vi "Send Trigger.vi"(8 "error in (no error)":errorcluster, 10 "Trigger Type (0: Bus)":u16(ring) items=["Bus", "Immediate"], 11 "VISA resource name":refnum<visa-resource-name>) -> (0 "error out":errorcluster, 3 "VISA resource name out":refnum<visa-resource-name>)   [LabVIEW 2017, in "HH PLI Series.lvlib"]
doc: "Sends a software based trigger.\n\n<b>Note</b>\nA \"Bus\" trigger produces a trigger event, if trigger source \"Bus\" is chosen.\nAn \"Immediate\" trigger produces a source-independent trigger event."
uses:
  HH PLI Series.lvlib
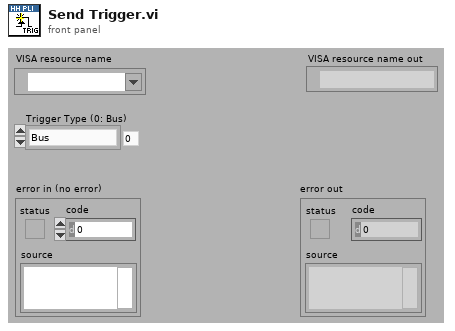
[diagram p1: front panel]
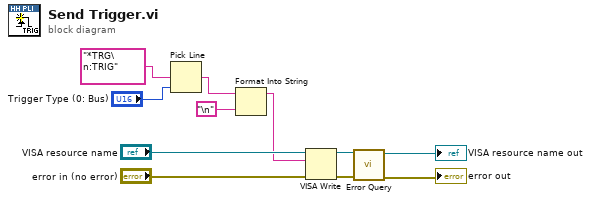
[diagram p0: block diagram]
diagram:
  n1 = Pick Line(multi-line string="*TRG\n:TRIG", line index="Trigger Type (0: Bus)") -> (output string=w2:string)  [unwired: 1 in]
  n2 = Format Into String(initial string=w2, "\n") -> (resulting string=w1:string)  [unwired: 2 in, 1 out]
  n3 = VISA Write(VISA resource name="VISA resource name", write buffer=w1, error in (no error)="error in (no error)") -> (VISA resource name out=w8:refnum<visa-resource-name>, error out=w9:errorcluster)  [unwired: 1 out]
  n4 = call "Error Query.vi"("error in (no error)"=w9, "VISA resource name"=w8) -> ("error out"=→"error out":errorcluster, "VISA resource name out"=→"VISA resource name out":refnum<visa-resource-name>)  [unwired: 6 in, 2 out]
